vi "testPassIndicator.vi"() -> ()   [LabVIEW 2013, in "No Object Control TestCase.lvclass"]
uses:
  No Object Control TestCase.lvclass
panel:
  out "Pass":bool=TRUE
  out "error out":errorcluster
  in  "error in (no error)":errorcluster
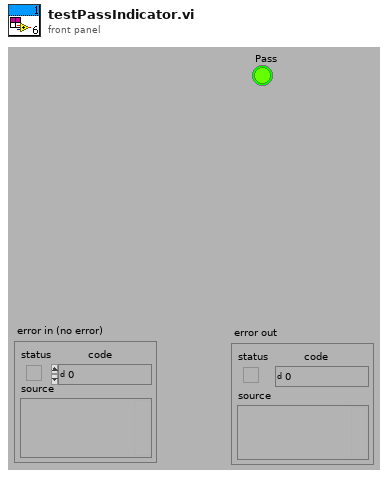
[diagram p1: front panel]
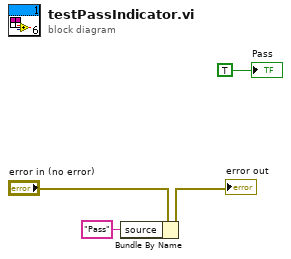
[diagram p0: block diagram]
diagram:
  n1 = Bundle By Name(cluster="error in (no error)", "source"="Pass") -> (→"error out":errorcluster)
  "Pass" <- TRUE
